vi "MTM2_putSample_zenithAngleMeasured.vi"(8 "error in (no error)":errorcluster, 11 "zenithAngleMeasured_Ctl":T1) -> (0 "error out":errorcluster, 2 "function return":i32, 3 "zenithAngleMeasured_Ctl out":T1)   [LabVIEW 2018, in "SALLV_MTM2.lvlib"]
doc: "int MTM2_shm_putSample_zenithAngleMeasuredLV(MTM2_zenithAngleMeasuredLV *zenithAngleMeasured_Ctl );"
uses:
  SALLV_MTM2.lvlib
  DataTypes/zenithAngleMeasured.ctl
  SALLV_MTM2.so
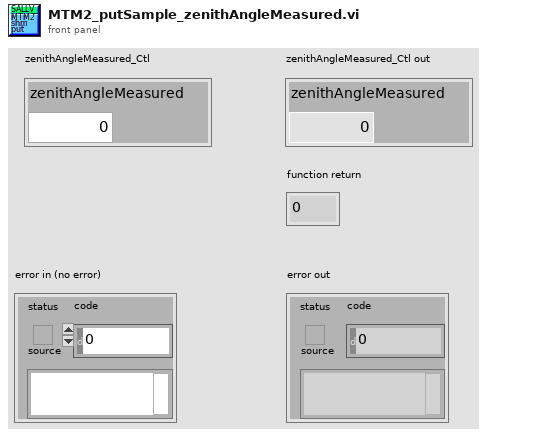
[diagram p1: front panel]
types:
  T1 = typedef "SALLV_MTM2.lvlib/zenithAngleMeasured.ctl" = cluster{"zenithAngleMeasured":dbl}
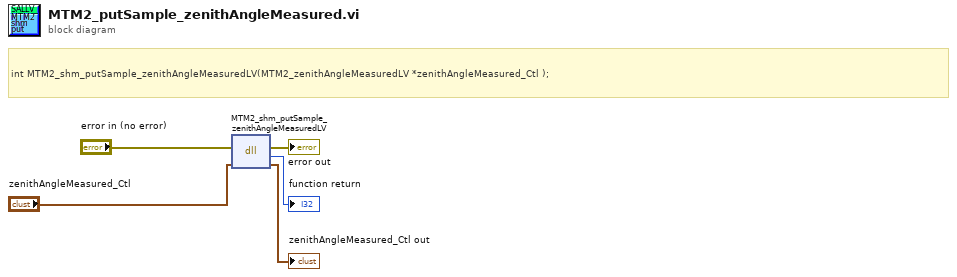
[diagram p0: block diagram]
diagram:
  # "int MTM2_shm_putSample_zenithAngleMeasuredLV(MTM2_zenithAngleMeasuredLV *zenithAngleMeasured_Ctl );"
  n1 = dll-call lib="home/ttsai/Document/salApiMTM2/SALLV_MTM2/SALLV_MTM2.*" fn="MTM2_shm_putSample_zenithAngleMeasuredLV"(error in="error in (no error)", "zenithAngleMeasured_Ctl"="zenithAngleMeasured_Ctl") -> (error out=→"error out":errorcluster, →"function return":i32, "zenithAngleMeasured_Ctl"=→"zenithAngleMeasured_Ctl out":T1)  [unwired: 2 in, 1 out]
